vi "libnodave_read_PLC.vi"(4 "length":i32=12, 5 "dataBlock":i32=31, 6 "start":i32, 7 "areaType":T1=132 items=["P Area"=128, "I Area"=129, "O Area"=130, "M Area"=131, "DB Area"=132, "Counter Area"=40, "Timer Area"=41], 8 "Error In":errorcluster, 9 "cpProtocol":i32=122, 10 "slot":i32=2, 11 "ip":string="172.18.214.231") -> (0 "Error Out":errorcluster, 1 "outBuffer":u8[](array[numeric]), 2 "logInfo":string, 3 "return":i32)   [LabVIEW 2014]
doc: "This VI makes uses of a C wrapper developed for the open-source libnodave library in order to read data from SIEMENS S-200, S-300 or S-400 PLCs."
uses:
  PLC_Libnodave_wrapper_areaType.ctl
  myDaveWrapper.dll
panel:
  # "RADE Libnodave PLC Read"
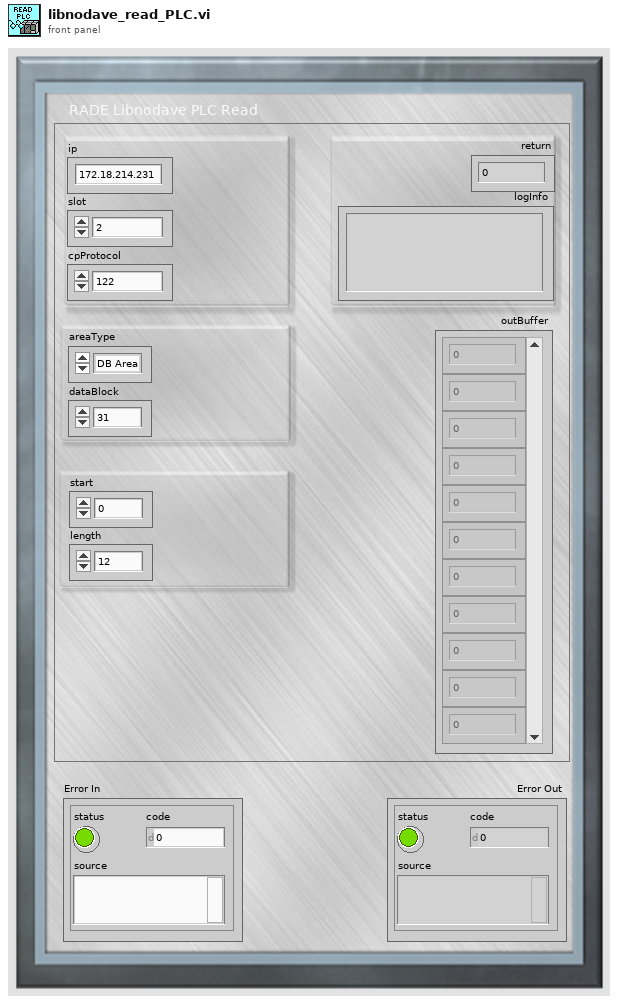
[diagram p1: front panel]
types:
  T1 = typedef "PLC_Libnodave_wrapper_areaType.ctl" = i32
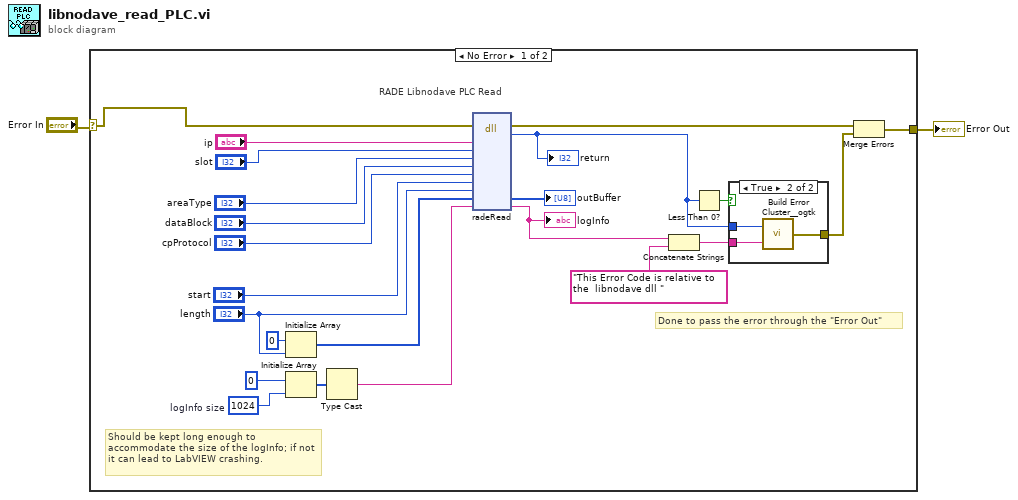
[diagram p0: block diagram]
diagram:
  n1 = case shown="No Error" "Error In" {
    selector: "Error In" -> [w3 w29]
    tunnel: [w5 w29] -> w1
    frame No Error {
      w19 = 1024  # logInfo size
      # "RADE Libnodave PLC Read"
      # "Done to pass the error through the \"Error Out\""
      # "Should be kept long enough to accommodate the size of the logInfo; if not it can lead to LabVIEW crashing."
      n2 = Initialize Array(u8 0, "length") -> (w6:u8[])
      n3 = Initialize Array(u8 0, w19) -> (w17:u8[])
      n4 = Type Cast(x=w17) -> (*(type *) &x=w16:string)  [unwired: 1 in]
      n5 = dll-call lib="C:/Users/coldex/Documents/COLDEX_LV_CG/trunk/Modules/PLC-libnodave/myDaveWrapper.dll" fn="radeRead"(error in=w3, "ip"="ip", "slot"="slot", "areaType"="areaType", "dataBlock"="dataBlock", "cpProtocol"="cpProtocol", "start"="start", "length"="length", "inBuffer"=w6, "logInfo"=w16) -> (error out=w4:errorcluster, "return"=w13:i32, "inBuffer"=→"outBuffer":u8[], "logInfo"=w10:string)  [unwired: 9 in, 1 out]
      "return" <- w13
      "logInfo" <- w10
      n6 = Concatenate Strings(w10, "This Error Code is relative to the  libnodave dll " ("string")) -> (w9:string)
      n7 = Less Than 0?(x=w13) -> (x < 0?=w14:bool)
      n8 = case shown="True" w14 {
        tunnel: w9 -> [_ w28]
        tunnel: w13 -> [_ w27]
        tunnel: [_ w26] -> w11
        frame False {
        }
        frame True {
          n9 = call <userlib>:"Build Error Cluster__ogtk.vi"("String to Prepend to source (\"\")"=w28, "code"=w27) -> ("error out"=w26:errorcluster)
        }
      }
      n10 = Merge Errors(w4, w11) -> (w5:errorcluster)
    }
    frame Error {
    }
  }
  "Error Out" <- w1
